vi "RT_DETR_OpenVINO_IR.vi"() -> ()   [LabVIEW 2018]
doc: "RT-DETR_OpenVINO_IR: This example is an object detection example of the RT-DETR algorithm, which can perform object detection on real-time images captured by cameras. IR is OpenVINO's proprietary optimized format model."
uses:
  vi.lib/VIRobotics/opencv_yiku/Cap/Cap.lvclass
  vi.lib/VIRobotics/ModelZoo/Object_Detection/RT_DETR_OpenVINO/RT_DETR_OpenVINO.lvclass
  vi.lib/VIRobotics/opencv_yiku/Mat/Mat_8U/Mat_8U.lvclass
panel:
  in  "config":T1={"confThreshold"=0.3, "nms_threshold"=0.5, "fontScale"=0.5}
  in  "device_name":string(combo)="CPU"
  in  "bin_fle":path=path "C:/ProgramData/VIRobotics/ModelZoo/Object_Detection/RT_DETR/IR_model/rtdetr_r50vd_m_6x_coco.bin"
  out "每帧耗时(s)":dbl
  in  "class_names_file":path=path "C:/ProgramData/VIRobotics/ModelZoo/Object_Detection/coco.names"
  in  "xml_file":path=path "C:/ProgramData/VIRobotics/ModelZoo/Object_Detection/RT_DETR/IR_model/rtdetr_r50vd_m_6x_coco.xml"
  in  "stop":bool
  out "picture":picture
  # "Overview: Demonstrates how to use OpenVINO to load the the IR model of pp-rtdetr for real-time object detection.\nRequirements: Windows.\nMake sure your computer has a camera。\nInstructions: \nIf you want to load the model, follow the following steps:\n1.Select the device_name to use.（If your computer has Intel GPU, you can select GPU in the \"type\" control before running the VI to achieve faster inference).\n2.Specify the xml_file、bin_file and class_names_file(Because the model is too large, it is not loaded by default.).\n3.Run the VI."
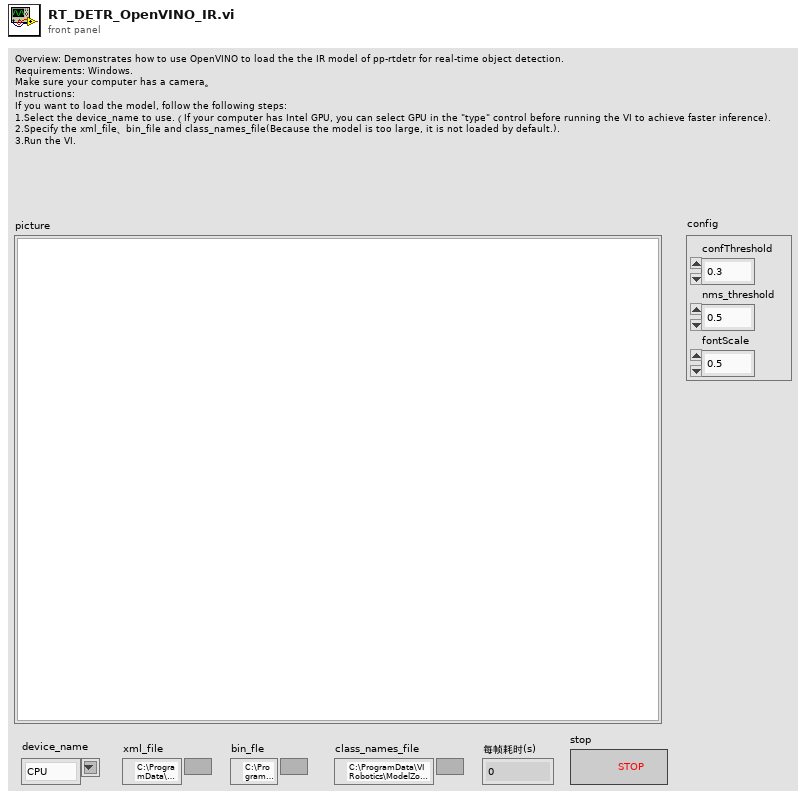
[diagram p1: front panel]
types:
  T1 = cluster{"confThreshold":sgl, "nms_threshold":sgl, "fontScale":dbl}
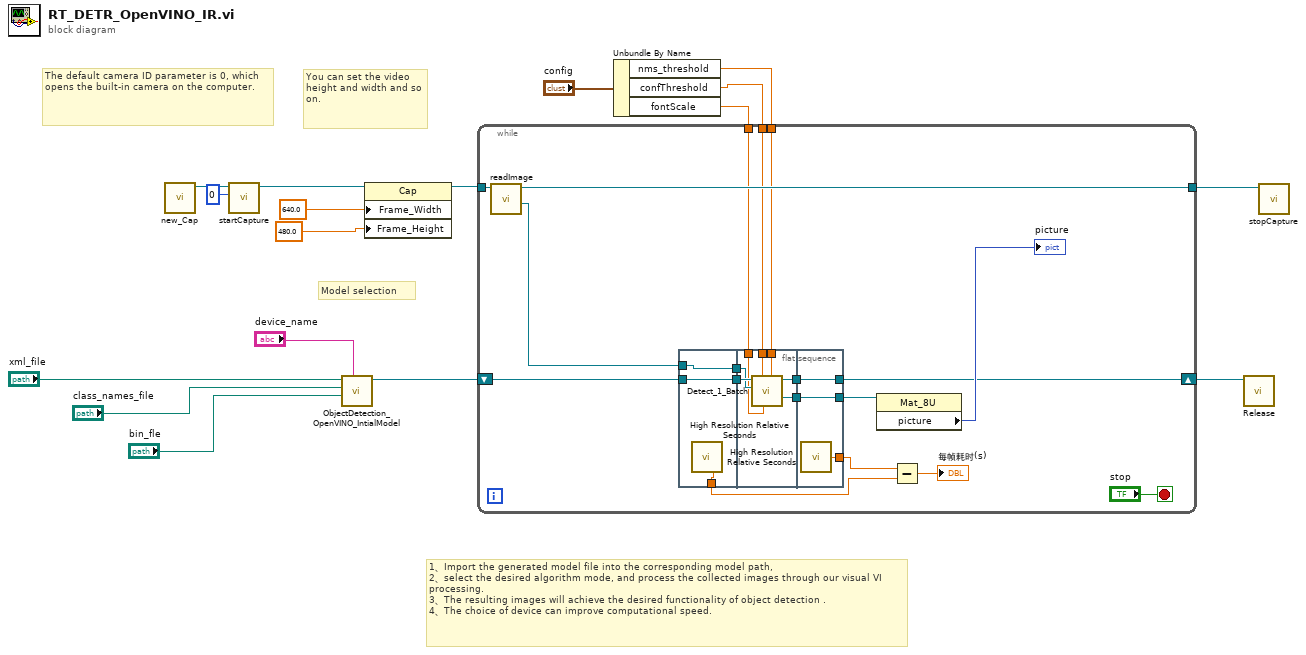
[diagram p0: block diagram]
diagram:
  # "1、Import the generated model file into the corresponding model path, \n2、select the desired algorithm mode, and process the collected images through our visual VI processing. \n3、The resulting images will achieve the desired functionality of object detection . \n4、The choice of device can improve computational speed."
  # "Model selection"
  # "You can set the video height and width and so on."
  # "The default camera ID parameter is 0, which opens the built-in camera on the computer."
  n1 = call "new_Cap.vi"() -> ("Cap out"=w10:refnum<class "Cap.lvclass">)  [unwired: 10 in, 1 out]
  n2 = call "startCapture.vi"("cameraID"=0, "Cap in"=w10) -> ("Cap out"=w9:refnum<class "Cap.lvclass">)  [unwired: 8 in, 1 out]
  n3 = call-poly "ObjectDetection_OpenVINO_IntialModel.vi"("device_name"="device_name", "bin_fle"="bin_fle", "class_names_path"="class_names_file", "xml file"="xml_file") -> ("detr_ov out"=w15:refnum<class "RT_DETR_OpenVINO.lvclass">)  [unwired: 6 in, 1 out]
  n4 = property class="Cap"(reference=w9, "Frame_Width"=640.0, "Frame_Height"=480.0) -> (reference out=w5:refnum<class "Cap.lvclass">)  [unwired: 1 in, 1 out]
  n5 = Unbundle By Name("config") -> ("nms_threshold"=w3:sgl, "confThreshold"=w2:sgl, "fontScale"=w1:dbl)
  n6 = while {
    tunnel: w5 -> [w34]
    shift-right: [w30] -> w16
    shift-left: w15 -> [w35]
    tunnel: [w29] -> w17
    tunnel: w3 -> [w20]
    tunnel: w2 -> [w19]
    tunnel: w1 -> [w18]
    stop <- "stop" stop-if-true
    n7 = call "readImage.vi"("Cap in"=w34) -> ("Mat out"=w22:refnum<class "Mat_8U.lvclass">, "Cap out"=w29:refnum<class "Cap.lvclass">)  [unwired: 8 in, 1 out]
    n8 = flat-sequence {
      tunnel: w35 -> [w38]
      tunnel: [w38] -> w28
      tunnel: [w37] -> w24
      tunnel: w22 -> [w36]
      tunnel: [w36] -> w21
      tunnel: w28 -> [w45]
      tunnel: [w44] -> w27
      tunnel: [w43] -> w26
      tunnel: w21 -> [w42]
      tunnel: w20 -> [w41]
      tunnel: w19 -> [w40]
      tunnel: w18 -> [w39]
      tunnel: [w47] -> w30
      tunnel: [w48] -> w33
      tunnel: w27 -> [w48]
      tunnel: w26 -> [w47]
      tunnel: [w46] -> w25
      frame #0 {
        n9 = call <vilib>:"High Resolution Relative Seconds.vi"() -> ("relative seconds"=w37:dbl)
      }
      frame #1 {
        n10 = call-dynamic "Detect_1_Batch.vi"("nms_threshold"=w41, "fontScale"=w39, "confThreshold"=w40, "image"=w42, "RT_DETR_OpenVINO in"=w45) -> ("img out"=w44:refnum<class "Mat_8U.lvclass">, "RT_DETR_OpenVINO out"=w43:refnum<class "RT_DETR_OpenVINO.lvclass">)  [unwired: 3 in, 2 out]
      }
      frame #2 {
        n11 = call <vilib>:"High Resolution Relative Seconds.vi"() -> ("relative seconds"=w46:dbl)
      }
    }
    n12 = property class="Mat_8U"(reference=w33) -> ("picture"=→"picture":picture)  [unwired: 1 in, 2 out]
    n13 = Subtract(x=w25, y=w24) -> (x-y=→"每帧耗时(s)":dbl)
  }
  n14 = call-dynamic "Release.vi"("RT_DETR_OpenVINO in"=w16) -> ()  [unwired: 9 in, 2 out]
  n15 = call "stopCapture.vi"("Cap in"=w17) -> ()  [unwired: 10 in, 1 out]
